vi "Graph by UT.vi"(8 "Ch":u16(ring) items=["Vin Ch 1", "Vin Ch 2", "Vin Ch 3", "Vin Ch 4", "Vin Ch 5", "Vin Ch 6", "Vin Ch 7", "Vin Ch 8", "Vin Ch 9", "Vin Ch 10", "Vout Ch 1", "Vout Ch 2", "Vout Ch 3", "Vout Ch 4", "Vout Ch 5", "Vout Ch 6", "Vout Ch 7", "Vout Ch 8", "Vout Ch 9", "Vout Ch 10", "Temp1", "Temp 2", "Curren Ch 1", "Curren Ch 2", "Curren Ch 3", "Curren Ch 4", "Curren Ch 5", "Curren Ch 6", "Curren Ch 7", "Curren Ch 8", "Curren Ch 9", "Curren Ch 10"], 10 "UnitType":T1(ring)) -> (0 "index":i32, 1 "ID":u32, 2 "Data 2":u8[](array[numeric]))   [LabVIEW 2017]
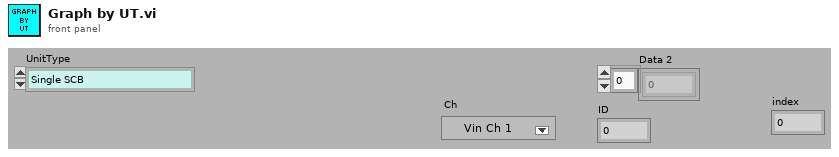
[diagram p1: front panel]
types:
  T1 = enum16{"Single SCB", "Power Rider", "Power Rider&Next10", "HATAL", "DAPH", "Indefinite"}
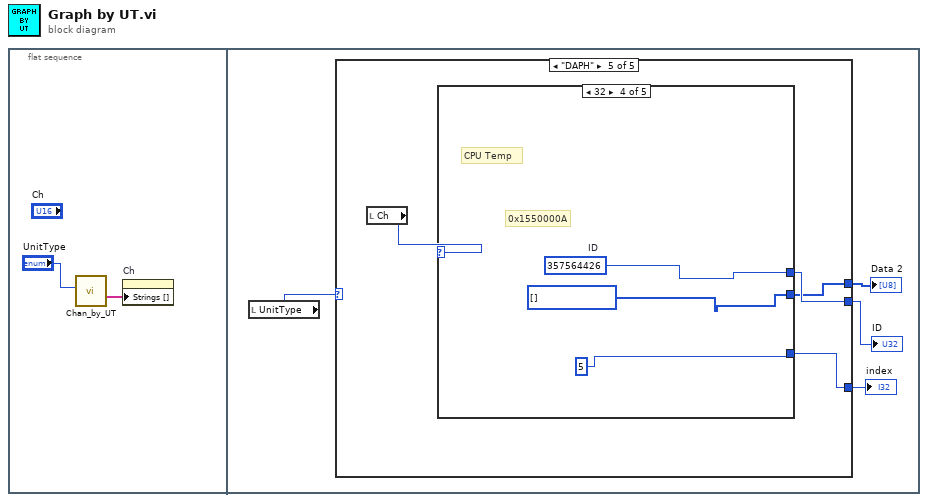
[diagram p0: block diagram]
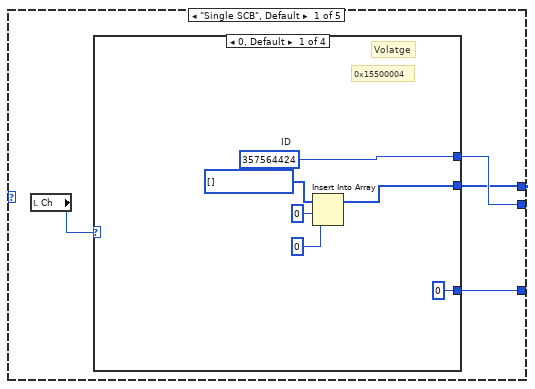
[diagram p2: hidden frame]
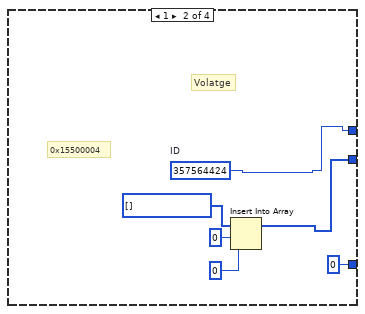
[diagram p3: hidden frame]
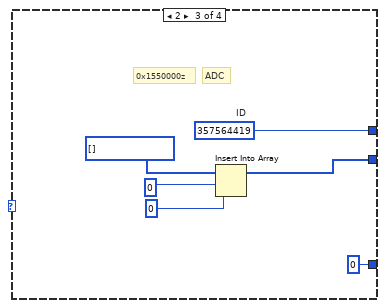
[diagram p4: hidden frame]
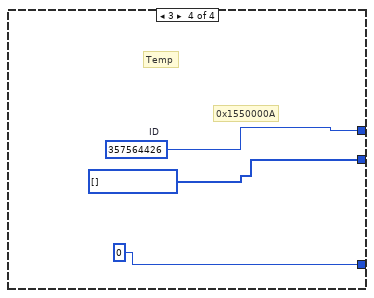
[diagram p5: hidden frame]
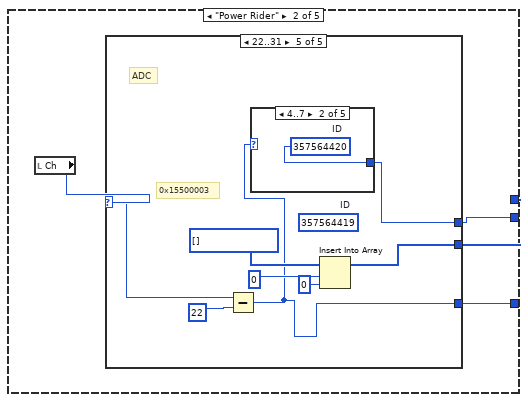
[diagram p6: hidden frame]
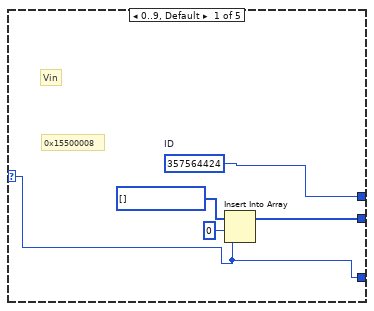
[diagram p7: hidden frame]
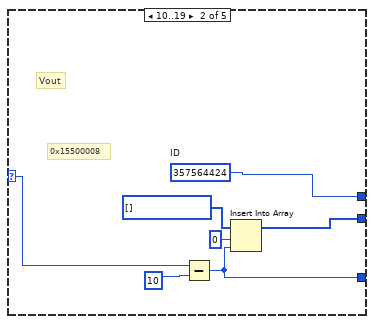
[diagram p8: hidden frame]
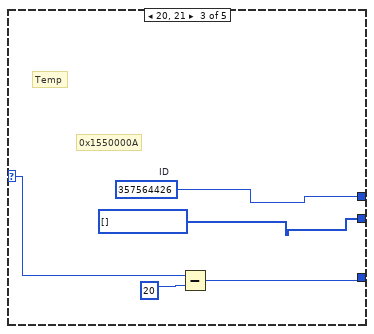
[diagram p9: hidden frame]
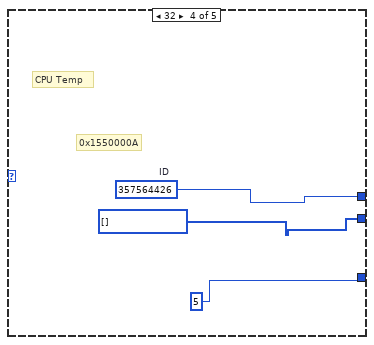
[diagram p10: hidden frame]
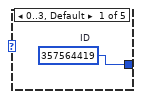
[diagram p11: hidden frame]
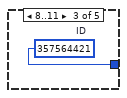
[diagram p12: hidden frame]
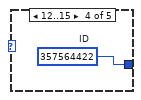
[diagram p13: hidden frame]
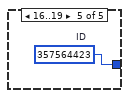
[diagram p14: hidden frame]
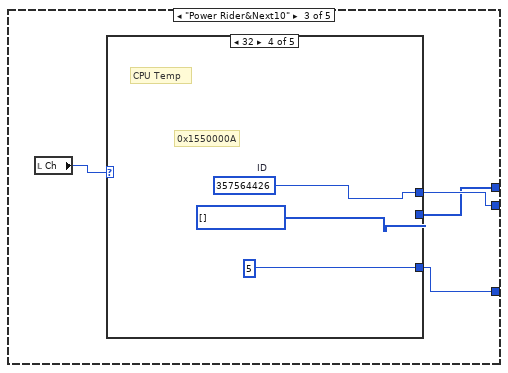
[diagram p15: hidden frame]
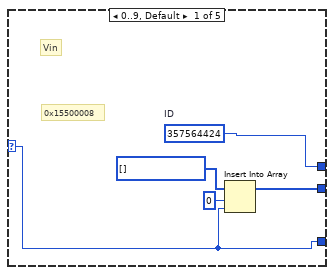
[diagram p16: hidden frame]
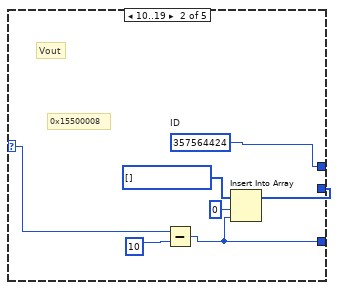
[diagram p17: hidden frame]
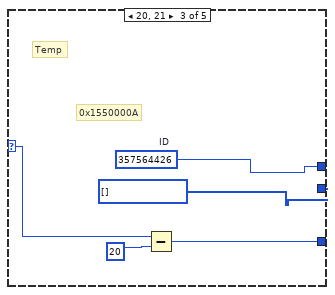
[diagram p18: hidden frame]
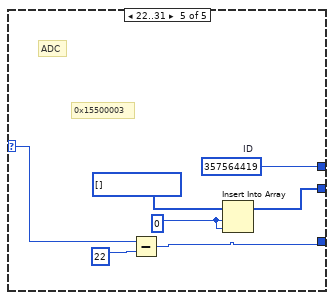
[diagram p19: hidden frame]
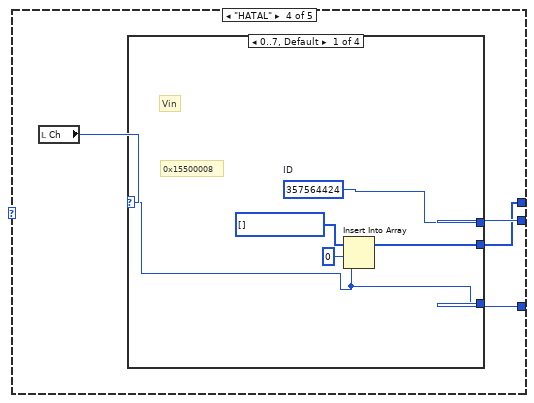
[diagram p20: hidden frame]
diagram:
  n1 = flat-sequence {
    frame #0 {
      n2 = call "Chan_by_UT.vi"("UnitType 2"="UnitType") -> ("Graph Strings [] 2"=w2:string[])  [unwired: 7 in, 1 out]
      n3 = property on="Ch" class="Ring (strict)"("Strings []"=w2) -> ()  [unwired: 2 in, 2 out]
    }
    frame #1 {
      n4 = local read "UnitType"() -> (w3:T1)
      n5 = case shown="\"DAPH\"" w3 {
        tunnel: [w10 w33 w71 w103 w134] -> w6
        tunnel: [w9 w35 w70 w100 w133] -> w5
        tunnel: [w7 w32 w69 w102 w135] -> w4
        frame "Single SCB", Default {
          n6 = local read "Ch"() -> (w8:u16)
          n7 = case shown="0, Default" w8 {
            tunnel: [w13 w18 w25 u8[] [] ("Data 2")] -> w9
            tunnel: [w12 w19 w24 w30] -> w10
            tunnel: [u16 0 ("y") u16 0 ("y") u16 0 ("y") u16 0 ("y")] -> w7
            frame 0, Default {
              w12 = u32 357564424  # ID
              # "Volatge"
              # "0x15500004"
              n8 = Insert Into Array(array=u8[] [] ("Data 2"), index=0, new element=u8 0 ("new element/subarray")) -> (w13:u8[])
            }
            frame 1 {
              w19 = u32 357564424  # ID
              # "Volatge"
              # "0x15500004"
              n9 = Insert Into Array(array=u8[] [] ("Data 2"), index=0, new element=u8 0 ("new element/subarray")) -> (w18:u8[])
            }
            frame 2 {
              w24 = u32 357564419  # ID
              # "ADC"
              # "0x1550000z"
              n10 = Insert Into Array(array=u8[] [] ("Data 2"), index=0, new element=u8 0 ("new element/subarray")) -> (w25:u8[])
            }
            frame 3 {
              w30 = u32 357564426  # ID
              # "Temp"
              # "0x1550000A"
            }
          }
        }
        frame "Power Rider" {
          n11 = local read "Ch"() -> (w34:u16)
          n12 = case shown="22..31" w34 {
            selector: w34 -> [w36 w42 w49 _ w60]
            tunnel: [w38 w45 u8[] [] ("Data 2") u8[] [] ("Data 2") w61] -> w35
            tunnel: [w37 w44 w52 w55 w58] -> w33
            tunnel: [w36 w41 w48 u16 5 ("y") w57] -> w32
            frame 0..9, Default {
              w37 = u32 357564424  # ID
              # "0x15500008"
              # "Vin"
              n13 = Insert Into Array(array=u8[] [] ("Data 2"), index=0, new element=w36) -> (w38:u8[])
            }
            frame 10..19 {
              w44 = u32 357564424  # ID
              # "Vout"
              # "0x15500008"
              n14 = Subtract(x=w42, y=u16 10) -> (x-y=w41:u16)
              n15 = Insert Into Array(array=u8[] [] ("Data 2"), index=0, new element=w41) -> (w45:u8[])
            }
            frame 20, 21 {
              w52 = u32 357564426  # ID
              # "Temp"
              # "0x1550000A"
              n16 = Subtract(x=w49, y=u16 20) -> (x-y=w48:u16)
            }
            frame 32 {
              w55 = u32 357564426  # ID
              # "CPU Temp"
              # "0x1550000A"
            }
            frame 22..31 {
              (unwired) u32 357564419  # ID
              # "ADC"
              # "0x15500003"
              n17 = Subtract(x=w60, y=u16 22) -> (x-y=w57:u16)
              n18 = case shown="4..7" w57 {
                tunnel: [w64 w65 w66 w67 w68] -> w58
                frame 0..3, Default {
                  w64 = u32 357564419  # ID
                }
                frame 4..7 {
                  w65 = u32 357564420  # ID
                }
                frame 8..11 {
                  w66 = u32 357564421  # ID
                }
                frame 12..15 {
                  w67 = u32 357564422  # ID
                }
                frame 16..19 {
                  w68 = u32 357564423  # ID
                }
              }
              n19 = Insert Into Array(array=u8[] [] ("Data 2"), index=0, new element=u8 0 ("new element/subarray")) -> (w61:u8[])
            }
          }
        }
        frame "Power Rider&Next10" {
          n20 = local read "Ch"() -> (w72:u16)
          n21 = case shown="32" w72 {
            selector: w72 -> [w73 w79 w86 _ w96]
            tunnel: [w75 w82 u8[] [] ("Data 2") u8[] [] ("Data 2") w97] -> w70
            tunnel: [w74 w81 w89 w92 w98] -> w71
            tunnel: [w73 w78 w85 u16 5 ("y") w94] -> w69
            frame 0..9, Default {
              w74 = u32 357564424  # ID
              # "0x15500008"
              # "Vin"
              n22 = Insert Into Array(array=u8[] [] ("Data 2"), index=0, new element=w73) -> (w75:u8[])
            }
            frame 10..19 {
              w81 = u32 357564424  # ID
              # "Vout"
              # "0x15500008"
              n23 = Subtract(x=w79, y=u16 10) -> (x-y=w78:u16)
              n24 = Insert Into Array(array=u8[] [] ("Data 2"), index=0, new element=w78) -> (w82:u8[])
            }
            frame 20, 21 {
              w89 = u32 357564426  # ID
              # "Temp"
              # "0x1550000A"
              n25 = Subtract(x=w86, y=u16 20) -> (x-y=w85:u16)
            }
            frame 32 {
              w92 = u32 357564426  # ID
              # "CPU Temp"
              # "0x1550000A"
            }
            frame 22..31 {
              w93 = 0 ("index")
              w98 = u32 357564419  # ID
              # "ADC"
              # "0x15500003"
              n26 = Subtract(x=w96, y=u16 22) -> (x-y=w94:u16)
              n27 = Insert Into Array(array=u8[] [] ("Data 2"), index=w93, new element=w93) -> (w97:u8[])
            }
          }
        }
        frame "HATAL" {
          n28 = local read "Ch"() -> (w101:u16)
          n29 = case shown="0..7, Default" w101 {
            selector: w101 -> [w104 w110 w117 w125]
            tunnel: [w106 w113 u8[] [] ("Data 2") w126] -> w100
            tunnel: [w105 w112 w120 w123] -> w103
            tunnel: [w104 w109 w116 w122] -> w102
            frame 0..7, Default {
              w105 = u32 357564424  # ID
              # "0x15500008"
              # "Vin"
              n30 = Insert Into Array(array=u8[] [] ("Data 2"), index=0, new element=w104) -> (w106:u8[])
            }
            frame 8..15 {
              w112 = u32 357564424  # ID
              # "Vout"
              # "0x15500008"
              n31 = Subtract(x=w110, y=u16 8) -> (x-y=w109:u16)
              n32 = Insert Into Array(array=u8[] [] ("Data 2"), index=0, new element=w109) -> (w113:u8[])
            }
            frame 16, 17 {
              w120 = u32 357564426  # ID
              # "Temp"
              # "0x1550000A"
              n33 = Subtract(x=w117, y=u16 16) -> (x-y=w116:u16)
            }
            frame 18..25 {
              w121 = 0 ("index")
              (unwired) u32 357564419  # ID
              # "ADC"
              # "0x15500003"
              n34 = Subtract(x=w125, y=u16 18) -> (x-y=w122:u16)
              n35 = case shown="4..7" w122 {
                tunnel: [w128 w129 w130 w131 w132] -> w123
                frame 0..3, Default {
                  w128 = u32 357564419  # ID
                }
                frame 4..7 {
                  w129 = u32 357564420  # ID
                }
                frame 8..11 {
                  w130 = u32 357564421  # ID
                }
                frame 12..15 {
                  w131 = u32 357564422  # ID
                }
                frame 16..19 {
                  w132 = u32 357564423  # ID
                }
              }
              n36 = Insert Into Array(array=u8[] [] ("Data 2"), index=w121, new element=w121) -> (w126:u8[])
            }
          }
        }
        frame "DAPH" {
          n37 = local read "Ch"() -> (w136:u16)
          n38 = case shown="32" w136 {
            selector: w136 -> [w137 w143 w150 _ w161]
            tunnel: [w139 w146 u8[] [] ("Data 2") u8[] [] ("Data 2") w162] -> w133
            tunnel: [w138 w145 w153 w156 w159] -> w134
            tunnel: [w137 w142 w149 u16 5 ("y") w158] -> w135
            frame 0..9, Default {
              w138 = u32 357564424  # ID
              # "0x15500008"
              # "Vin"
              n39 = Insert Into Array(array=u8[] [] ("Data 2"), index=0, new element=w137) -> (w139:u8[])
            }
            frame 10..19 {
              w145 = u32 357564424  # ID
              # "Vout"
              # "0x15500008"
              n40 = Subtract(x=w143, y=u16 10) -> (x-y=w142:u16)
              n41 = Insert Into Array(array=u8[] [] ("Data 2"), index=0, new element=w142) -> (w146:u8[])
            }
            frame 20, 21 {
              w153 = u32 357564426  # ID
              # "Temp"
              # "0x1550000A"
              n42 = Subtract(x=w150, y=u16 20) -> (x-y=w149:u16)
            }
            frame 32 {
              w156 = u32 357564426  # ID
              # "CPU Temp"
              # "0x1550000A"
            }
            frame 22..31 {
              w157 = 0 ("index")
              (unwired) u32 357564419  # ID
              # "ADC"
              # "0x15500003"
              n43 = Subtract(x=w161, y=u16 22) -> (x-y=w158:u16)
              n44 = case shown="4..7" w158 {
                tunnel: [w164 w165 w166 w167 w168] -> w159
                frame 0..3, Default {
                  w164 = u32 357564419  # ID
                }
                frame 4..7 {
                  w165 = u32 357564420  # ID
                }
                frame 8..11 {
                  w166 = u32 357564421  # ID
                }
                frame 12..15 {
                  w167 = u32 357564422  # ID
                }
                frame 16..19 {
                  w168 = u32 357564423  # ID
                }
              }
              n45 = Insert Into Array(array=u8[] [] ("Data 2"), index=w157, new element=w157) -> (w162:u8[])
            }
          }
        }
      }
      "Data 2" <- w5
      "ID" <- w6
      "index" <- w4
    }
  }
